vi "read station hall config.vi"(8 "error in":errorcluster, 11 "configuration file path in":path) -> (0 "error out":errorcluster, 1 "Motor Drift Compensation":i32[](array[numeric])=[25, 25, 25, 25, 25, 25, 25, 25], 2 "Hall Positions":i32[](array[numeric]), 3 "configuration file path out":path)   [LabVIEW 2018]
uses:
  05.UserVI's/file io/ini/type defs/ini file actions.ctl
  05.UserVI's/file io/ini/type defs/ini entry value.ctl
  05.UserVI's/file io/ini/type defs/ini entry types.ctl
  05.UserVI's/file io/ini/type defs/ini entry.ctl
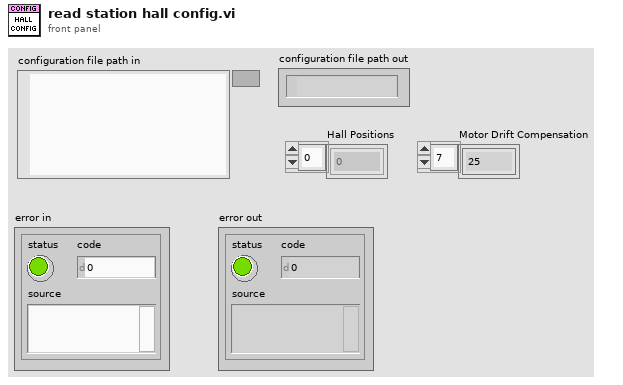
[diagram p1: front panel]
types:
  T1 = typedef "ini entry value.ctl" = cluster{"Boolean":bool, "Dbl":dbl, "I32":i32, "Path":path, "String":string, "U32":u32}
  T2 = typedef "ini file actions.ctl" = enum16{"read ini", "write ini"}
  T3 = typedef "ini entry.ctl" = cluster{"section":string, "key":string, "type":T4, "default value":T1}
  T4 = typedef "ini entry types.ctl" = enum16{"Boolean", "Double", "I32", "Path", "String", "U32"}
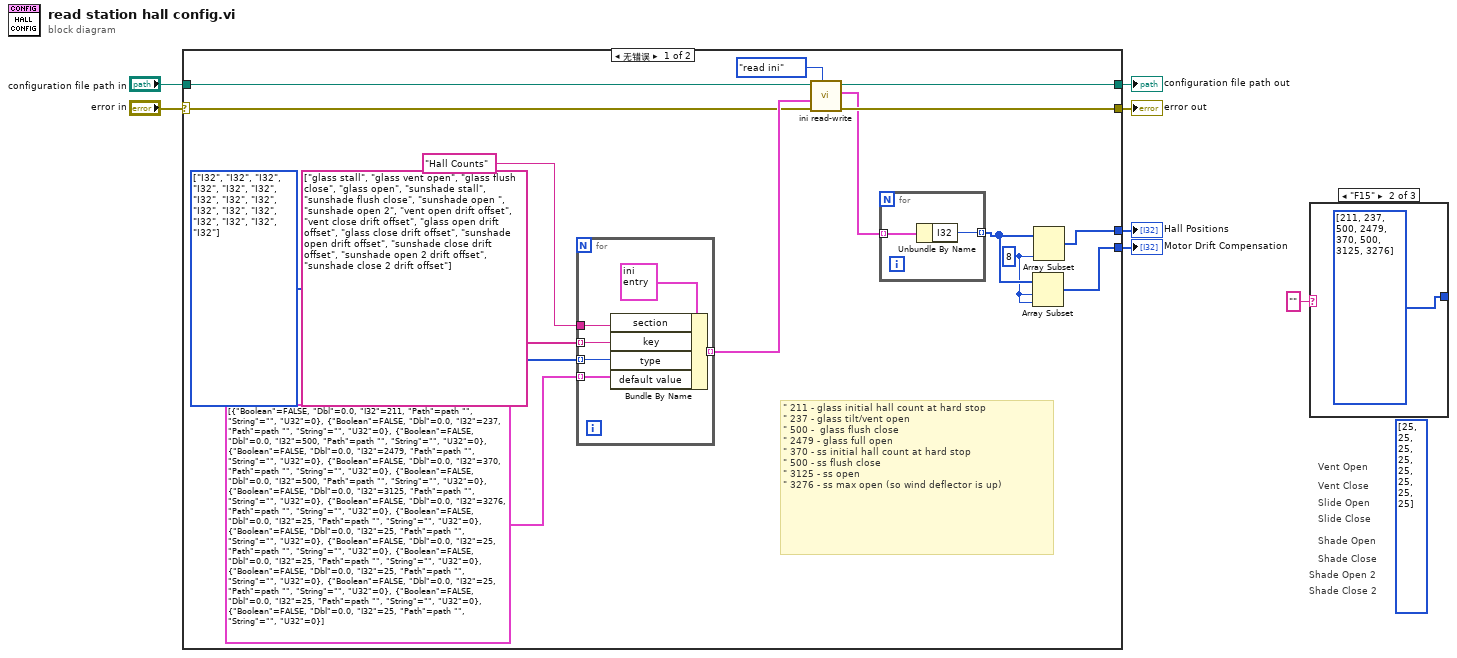
[diagram p0: block diagram]
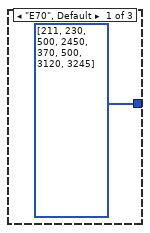
[diagram p2: hidden frame]
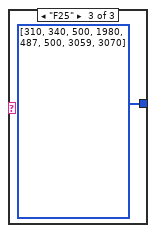
[diagram p3: hidden frame]
diagram:
  (unwired) i32[] [25, 25, 25, 25, 25, 25, 25, 25] ("Motor Drift Compensation")
  # "Shade Close 2"
  # "Shade Open 2"
  # "Shade Close"
  # "Shade Open"
  # "Slide Close"
  # "Slide Open"
  # "Vent Close"
  # "Vent Open"
  n1 = case shown="无错误" "error in" {
    selector: "error in" -> [w15 w32]
    tunnel: "configuration file path in" -> [w22 w31]
    tunnel: [w20 w31] -> w6
    tunnel: [w14 w32] -> w5
    tunnel: [w10 _] -> w2
    tunnel: [w9 _] -> w1
    frame No Error {
      w11 = 8 ("length")
      w18 = T4[] [enum."I32", enum."I32", enum."I32", enum."I32", enum."I32", enum."I32", enum."I32", enum."I32", enum."I32", enum."I32", enum."I32", enum."I32", enum."I32", enum."I32", enum."I32", enum."I32"] items=["Boolean", "Double", "I32", "Path", "String", "U32"]
      # "\"\t211 - glass initial hall count at hard stop\n\"\t237 - glass tilt/vent open\n\"\t500 -  glass flush close\n\"\t2479 - glass full open\n\"\t370 - ss initial hall count at hard stop\n\"\t500 - ss flush close\n\" 3125 - ss open\n\"\t3276 - ss max open (so wind deflector is up)"
      n2 = for {
        tunnel: "Hall Counts" ("string") -> [w29]
        tunnel: string[] ["glass stall", "glass vent open", "glass flush close", "glass open", "sunshade stall", "sunshade flush close", "sunshade open ", "sunshade open 2", "vent open drift offset", "vent close drift offset", "glass open drift offset", "glass close drift offset", "sunshade open drift offset", "sunshade close drift offset", "sunshade open 2 drift offset", "sunshade close 2 drift offset"] -> [w28] mode=indexing
        tunnel: w18 -> [w27] mode=indexing
        tunnel: T1[] [{"Boolean"=FALSE, "Dbl"=0.0, "I32"=211, "Path"=path "", "String"="", "U32"=0}, {"Boolean"=FALSE, "Dbl"=0.0, "I32"=237, "Path"=path "", "String"="", "U32"=0}, {"Boolean"=FALSE, "Dbl"=0.0, "I32"=500, "Path"=path "", "String"="", "U32"=0}, {"Boolean"=FALSE, "Dbl"=0.0, "I32"=2479, "Path"=path "", "String"="", "U32"=0}, {"Boolean"=FALSE, "Dbl"=0.0, "I32"=370, "Path"=path "", "String"="", "U32"=0}, {"Boolean"=FALSE, "Dbl"=0.0, "I32"=500, "Path"=path "", "String"="", "U32"=0}, {"Boolean"=FALSE, "Dbl"=0.0, "I32"=3125, "Path"=path "", "String"="", "U32"=0}, {"Boolean"=FALSE, "Dbl"=0.0, "I32"=3276, "Path"=path "", "String"="", "U32"=0}, {"Boolean"=FALSE, "Dbl"=0.0, "I32"=25, "Path"=path "", "String"="", "U32"=0}, {"Boolean"=FALSE, "Dbl"=0.0, "I32"=25, "Path"=path "", "String"="", "U32"=0}, {"Boolean"=FALSE, "Dbl"=0.0, "I32"=25, "Path"=path "", "String"="", "U32"=0}, {"Boolean"=FALSE, "Dbl"=0.0, "I32"=25, "Path"=path "", "String"="", "U32"=0}, {"Boolean"=FALSE, "Dbl"=0.0, "I32"=25, "Path"=path "", "String"="", "U32"=0}, {"Boolean"=FALSE, "Dbl"=0.0, "I32"=25, "Path"=path "", "String"="", "U32"=0}, {"Boolean"=FALSE, "Dbl"=0.0, "I32"=25, "Path"=path "", "String"="", "U32"=0}, {"Boolean"=FALSE, "Dbl"=0.0, "I32"=25, "Path"=path "", "String"="", "U32"=0}] -> [w26] mode=indexing
        tunnel: [w25] -> w16 mode=indexing
        n3 = Bundle By Name(cluster=T3 {"section"="", "key"="", "type"=enum."Boolean", "default value"={"Boolean"=FALSE, "Dbl"=0.0, "I32"=0, "Path"=path "", "String"="", "U32"=0}}, "section"=w29, "key"=w28, "type"=w27, "default value"=w26) -> (w25:T3)
      }
      n4 = call "ini read-write.vi"("action"=ini_file_actions."read ini", "error in (no error)"=w15, "ini entry descriptors"=w16, "configuration file path"=w22) -> ("error out"=w14:errorcluster, "values out"=w13:T1[], "configuration file path out"=w20:path)  [unwired: 5 in]
      n5 = for {
        tunnel: w13 -> [w24] mode=indexing
        tunnel: [w23] -> w12 mode=indexing
        n6 = Unbundle By Name(w24) -> ("I32"=w23:i32)
      }
      n7 = Array Subset(array=w12, index=w11, length=w11) -> (w9:i32[])
      n8 = Array Subset(array=w12, length=w11) -> (w10:i32[])  [unwired: 1 in]
    }
    frame Error {
    }
  }
  "configuration file path out" <- w6
  "error out" <- w5
  "Hall Positions" <- w2
  "Motor Drift Compensation" <- w1
  n9 = case shown="\"F15\"" "" {
    tunnel: [i32[] [211, 230, 500, 2450, 370, 500, 3120, 3245] ("Hall Positions") i32[] [211, 237, 500, 2479, 370, 500, 3125, 3276] ("Hall Positions") i32[] [310, 340, 500, 1980, 487, 500, 3059, 3070] ("Hall Positions")] -> _
    frame "E70", Default {
    }
    frame "F15" {
    }
    frame "F25" {
    }
  }
